vi "Record_Initialize.vi"(8 "error in":errorcluster, 9 "First Image in":T1 {"Frame Data"."Image Type" items=["Grayscale (U8)", "Grayscale (I16)", "Grayscale (SGL)", "Complex (CSG)", "RGB (U32)", "HSL (U32)", "RGB (U64)", "Grayscale (U16)"]}, 10 "Settings in":T6={"Harware Configuration"={"Camera"="cam1", "Frames Per Second"=15, "Simulate Recording"=FALSE, "Simulated Recording Sample"=path "", "Timestamp Method"=enum."Camera Timestamp"}, "Base Recording Path"=path "", "Type Of Recording"="", "Recording Codec"="", "TrackingSettings"={"Max Radius"=0, "Threshold"=160.0, "ROI"={"Left"=0, "Top"=0, "Right"=0, "Bottom"=0, "Rotation"=0.0}}, "Calibration"={"Pixel Width (X)"=1.0, "Pixel Height (Y)"=1.0}, "Broadcast Length"=0} {"Broadcast Length" min=0; "TrackingSettings"."ROI"."Rotation" format="%.2f"; "TrackingSettings"."ROI"."Left" scale=0.0..1024.0; "TrackingSettings"."ROI"."Right" scale=0.0..1024.0; "TrackingSettings"."Threshold" scale=0.0..255.0}, 11 "Recording Data":T3) -> (0 "error out":errorcluster, 3 "Recording Data Out":T3)   [LabVIEW 2017, in "ImageAcquisitionLibrary.lvlib"]
uses:
  ImageAcquisitionLibrary.lvlib
  Settings/Settings.ctl
  <vilib>/userdefined/High Color/IMAQdx.ctl
  Tracking/TrackingSettings.ctl
  Settings/Calibration.ctl
  RecordingData.ctl
  <vilib>/vision/Image Controls.llb/IMAQ Image.ctl
  <vilib>/vision/Avi.llb/IMAQ AVI2 Refnum.ctl
  Acquisition/AcquireData.ctl
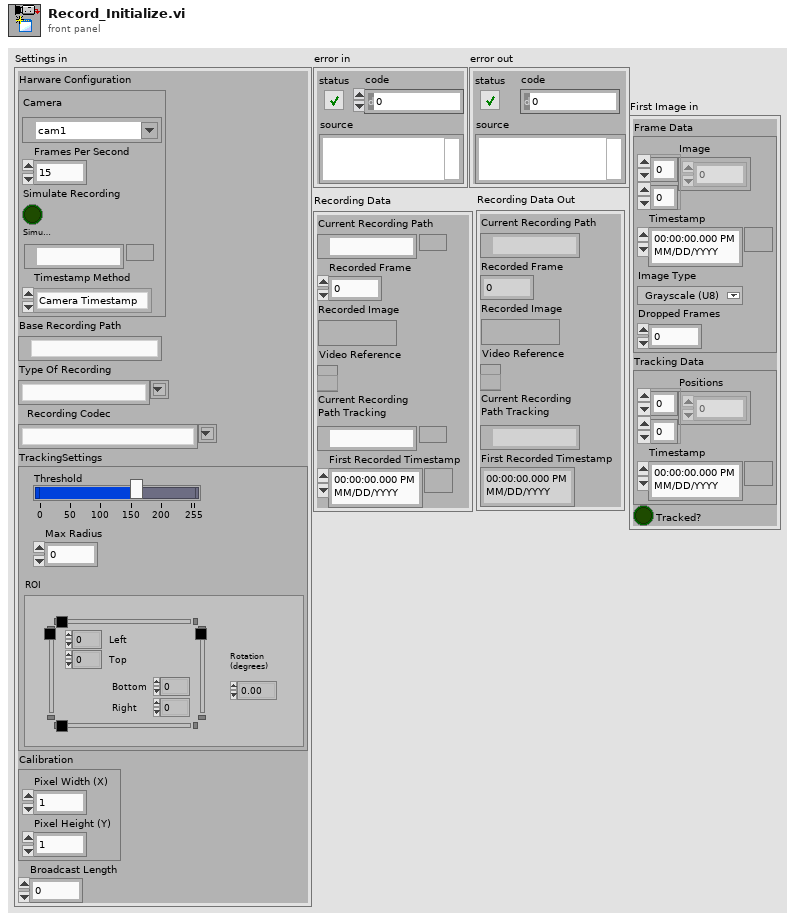
[diagram p1: front panel]
types:
  T1 = typedef "ImageAcquisitionLibrary.lvlib/AcquireData.ctl" = cluster{"Frame Data":cluster{"Image":u32[][], "Timestamp":timestamp, "Image Type":T2, "Dropped Frames":u32}, "Tracking Data":cluster{"Positions":dbl[][], "Timestamp":timestamp}, "Tracked?":bool}
  T2 = typedef "Image Type" = u32
  T3 = typedef "ImageAcquisitionLibrary.lvlib/RecordingData.ctl" = cluster{"Current Recording Path":path, "Recorded Frame":i32, "Recorded Image":T4, "Video Reference":T5, "Current Recording \nPath Tracking":path, "First Recorded Timestamp":timestamp}
  T4 = typedef "IMAQ Image.ctl" = refnum<image>
  T5 = typedef "IMAQ AVI2 Refnum.ctl" = refnum<k20>
  T6 = typedef "ImageAcquisitionLibrary.lvlib/Settings.ctl" = cluster{"Harware Configuration":cluster{"Camera":T7, "Frames Per Second":u32, "Simulate Recording":bool, "Simulated Recording Sample":path, "Timestamp Method":enum16{"System Timestamp", "Camera Timestamp", "IMAQdx Timestamp"}}, "Base Recording Path":path, "Type Of Recording":string, "Recording Codec":string, "TrackingSettings":T8, "Calibration":T10, "Broadcast Length":i32}
  T7 = typedef "IMAQdx.ctl" = refnum<k21>
  T8 = typedef "ImageAcquisitionLibrary.lvlib/TrackingSettings.ctl" = cluster{"Max Radius":i32, "Threshold":sgl, "ROI":T9}
  T9 = typedef "IMAQ Rectangle" = cluster{"Left":i32, "Top":i32, "Right":i32, "Bottom":i32, "Rotation":dbl}
  T10 = typedef "ImageAcquisitionLibrary.lvlib/Calibration.ctl" = cluster{"Pixel Width (X)":dbl, "Pixel Height (Y)":dbl}
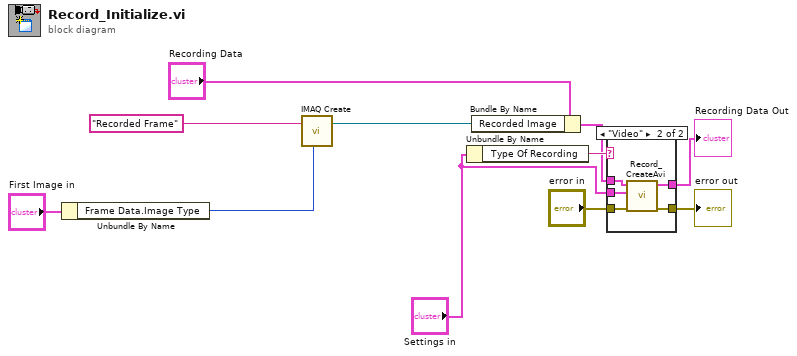
[diagram p0: block diagram]
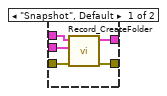
[diagram p2: hidden frame]
diagram:
  n1 = Unbundle By Name("First Image in") -> ("Frame Data.Image Type"=w1:T2)
  n2 = call "IMAQ Create"("Image Name"="Recorded Frame", "Image Type"=w1) -> ("New Image"=w5:T4)  [unwired: 3 in, 1 out]
  n3 = Unbundle By Name("Settings in") -> ("Type Of Recording"=w11:string)
  n4 = Bundle By Name(cluster="Recording Data", "Recorded Image"=w5) -> (w3:T3)
  n5 = case shown="\"Video\"" w11 {
    tunnel: w3 -> [w16 w21]
    tunnel: "error in" -> [w15 w20]
    tunnel: [w14 w19] -> w9
    tunnel: [w13 w18] -> w8
    tunnel: "Settings in" -> [w12 w17]
    frame "Snapshot", Default {
      n6 = call "Record_CreateFolder.vi"("error in"=w15, "Settings in"=w12, "Recording Data"=w16) -> ("error out"=w14:errorcluster, "Recording Data Out"=w13:T3)  [unwired: 7 in]
    }
    frame "Video" {
      n7 = call "Record_CreateAvi.vi"("error in"=w20, "Settings in"=w17, "Recording Data In"=w21) -> ("error out"=w19:errorcluster, "Recording Data Out"=w18:T3)  [unwired: 7 in]
    }
  }
  "error out" <- w9
  "Recording Data Out" <- w8
